vi "close.vi"(8 "error in (no error)":errorcluster, 11 "Lakeshore 331 in":refnum<class "Lakeshore 331.lvclass">) -> (0 "error out":errorcluster, 3 "Lakeshore 331 out":refnum<class "Lakeshore 331.lvclass">)   [LabVIEW 2022 SP3, in "Lakeshore 331.lvclass"]
uses:
  Lakeshore 331.lvclass
  Lakeshore 331.lvclass/Lakeshore 331.ctl
  Temp Control.lvclass
  <instrlib>/Lake Shore Cryotronics 331/Lake Shore Cryotronics 331.lvlib
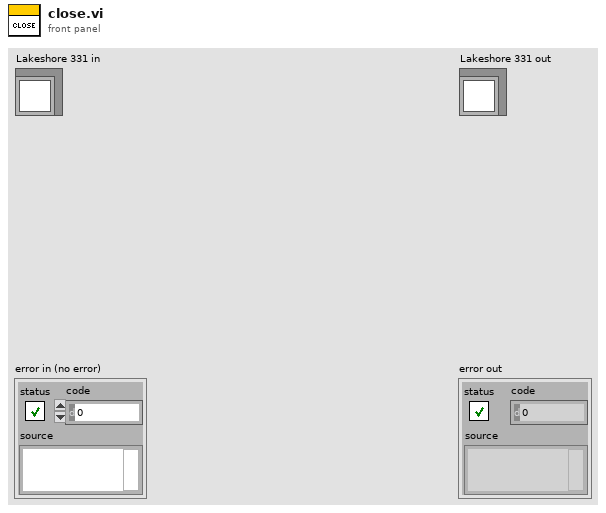
[diagram p1: front panel]
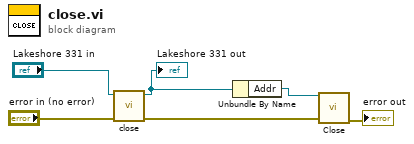
[diagram p0: block diagram]
diagram:
  n1 = call-parent <instrlib>:"close.vi"("error in (no error)"="error in (no error)", "Temp Control in"="Lakeshore 331 in") -> ("error out"=w2:errorcluster, "Temp Control out"=w4:refnum<class "Lakeshore 331.lvclass">)  [unwired: 8 in]
  "Lakeshore 331 out" <- w4
  n2 = Unbundle By Name(w4) -> ("Addr"=w3:refnum<visa-resource-name>)
  n3 = call <instrlib>:"Close.vi"("VISA resource name"=w3, "error in (no error)"=w2) -> ("error out"=→"error out":errorcluster)  [unwired: 13 in]
